vi "LiveVideo.vi"() -> ()   [LabVIEW 2019]
uses:
  <vilib>/userDefined/High Color/IMAQdx.ctl
  <vilib>/vision/driver/NI_Vision_Acquisition_Software.lvlib
  <vilib>/vision/NI_Vision_Development_Module.lvlib
panel:
  in  "Draw50umCircleAtCenter":bool
  out "Gcode":string
  in  "GetGantryXYZ":bool
  out "Position_XYZ":string
  in  "Corsshair":bool=TRUE
  out "Blue":T1(plugin-control)
  out "Green":T1(plugin-control)
  out "Red":T1(plugin-control)
  out "error out":errorcluster
  in  "Stop Button":bool
  out "Image":T1(plugin-control)
  in  "error in (no error)":errorcluster
  in  "Camera":T2="cam1"
  in  "ImageName":string="name1"
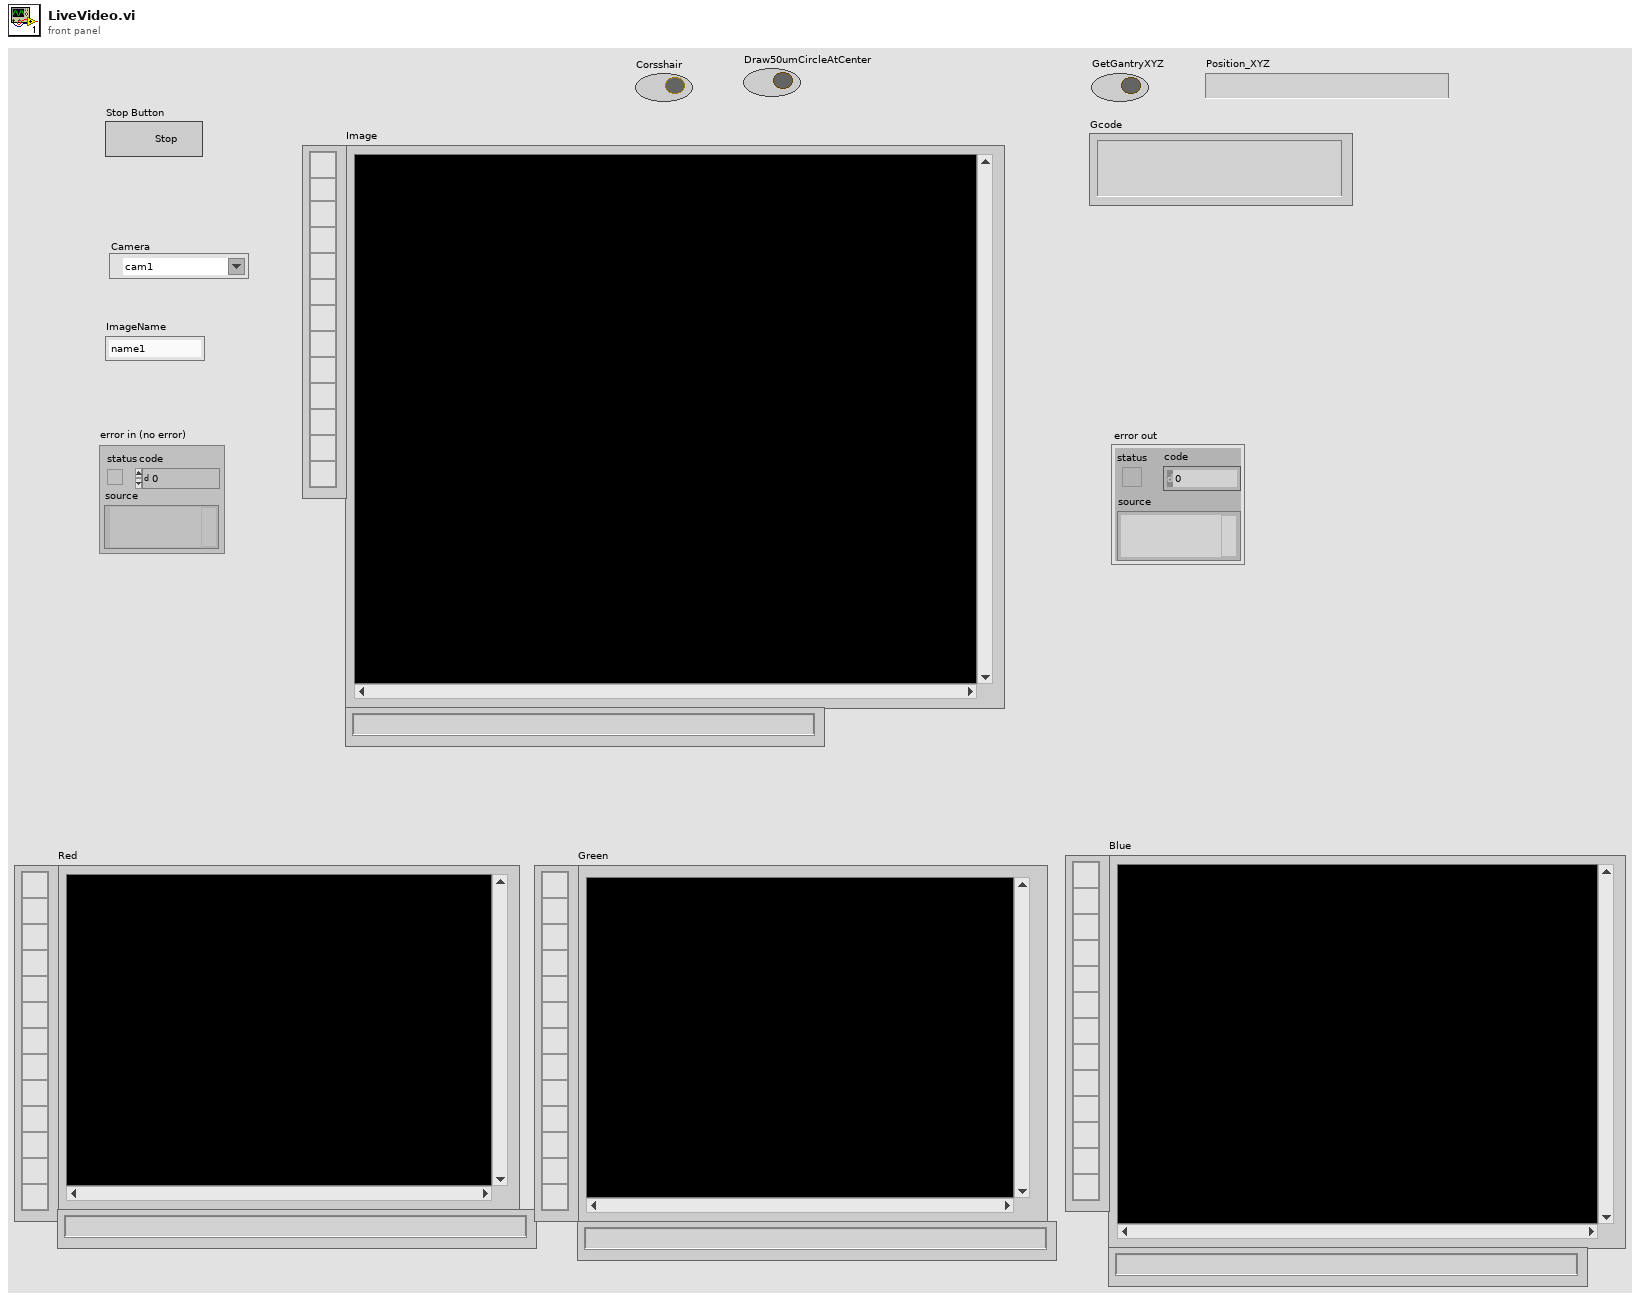
[diagram p1: front panel]
types:
  T1 = typedef "IMAQ Image.ctl" = refnum<image>
  T2 = typedef "IMAQdx.ctl" = refnum<k21>
  T3 = typedef "IMAQ Circle" = cluster{"Center X":i32, "Center Y":i32, "Inner Radius":i32, "Outer Radius":i32, "Start Angle":dbl, "End Angle":dbl}
  T4 = typedef "Image Type" = u32
  T5 = typedef "ROI Descriptor" = cluster{"Global Rectangle":i32[], "Contours":cluster{"ID":enum32{"External", "Internal"}, "Type":u32, "Coordinates":i32[]}[]}
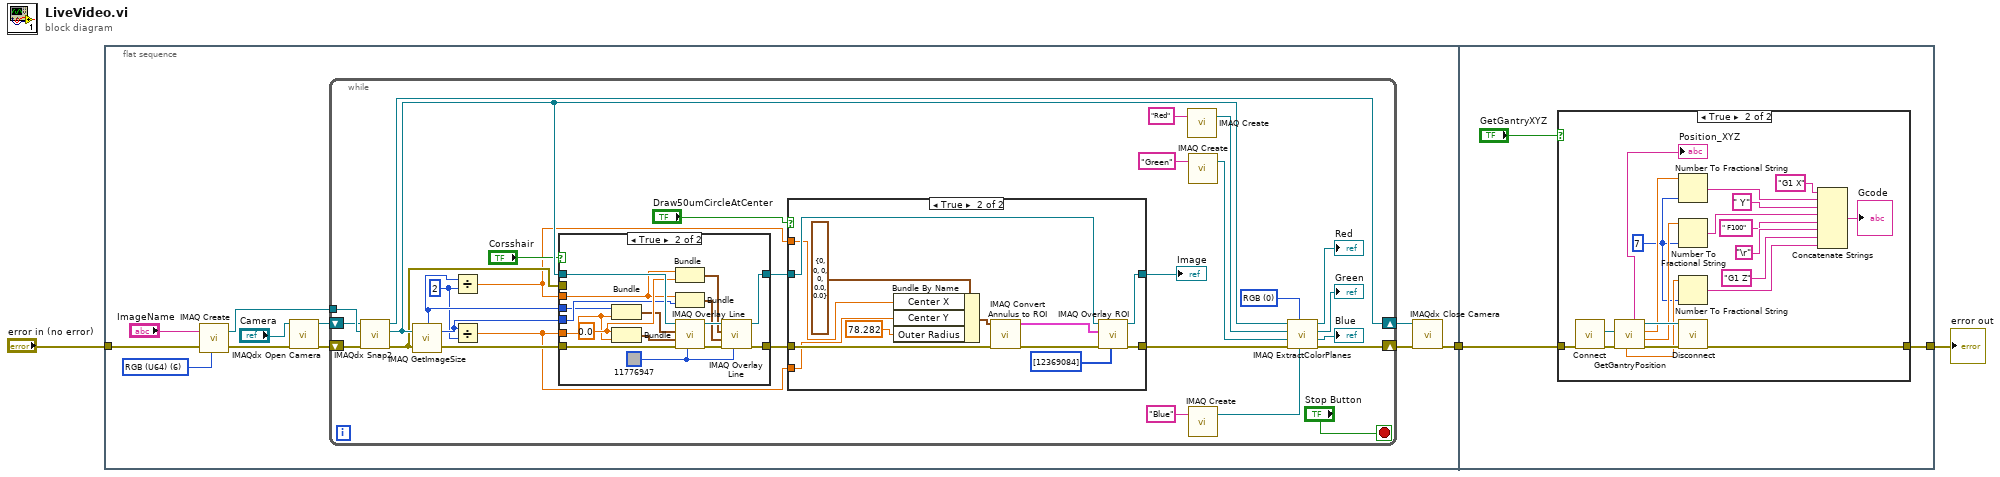
[diagram p0: block diagram]
diagram:
  n1 = flat-sequence {
    tunnel: "error in (no error)" -> [w10]
    tunnel: [w4] -> w2
    tunnel: w2 -> [w78]
    tunnel: [w77] -> w1
    frame #0 {
      w5 = T4 6 items=["Grayscale (U8)", "Grayscale (I16)", "Grayscale (SGL)", "Complex (CSG)", "RGB (U32)", "HSL (U32)", "RGB (U64)", "Grayscale (U16)"] ("Image Type")
      n2 = call "IMAQ Create"("Image Name"="ImageName", "Image Type"=w5, "error in (no error)"=w10) -> ("New Image"=w6:T1, "error out"=w7:errorcluster)  [unwired: 2 in]
      n3 = call <vilib>:"IMAQdx Open Camera.vi"("error in"=w7, "Session In"="Camera") -> ("error out"=w12:errorcluster, "Session Out"=w13:T2)  [unwired: 8 in]
      n4 = while {
        tunnel: w6 -> [w44]
        shift-right: [w27] -> w14
        shift-left: w12 -> [w42]
        shift-right: [w43] -> w11
        shift-left: w13 -> [w41]
        stop <- "Stop Button" stop-if-true
        w16 = 2 ("y")
        w38 = u16 0 items=["RGB", "HSL", "HSV", "HSI"] ("Color Mode")
        n5 = call <vilib>:"IMAQdx Snap2.vi"("error in"=w42, "Image In"=w44, "Session In"=w41) -> ("error out"=w28:errorcluster, "Image Out"=w29:T1, "Session Out"=w43:T2)  [unwired: 6 in]
        n6 = call "IMAQ GetImageSize"("Image"=w29, "error in (no error)"=w28) -> ("Y Resolution"=w20:i32, "X Resolution"=w19:i32, "error out"=w18:errorcluster)  [unwired: 2 in]
        n7 = Divide(x=w19, y=w16) -> (x/y=w15:dbl)
        n8 = Divide(x=w20, y=w16) -> (x/y=w17:dbl)
        n9 = case shown="True" "Corsshair" {
          tunnel: w29 -> [w60 w76]
          tunnel: w28 -> [w59 _]
          tunnel: [w60 w67] -> w25
          tunnel: [w59 w66] -> w24
          tunnel: w20 -> [_ w65]
          tunnel: w19 -> [_ w64]
          tunnel: w18 -> [_ w63]
          tunnel: w17 -> [_ w62]
          tunnel: w15 -> [_ w61]
          frame False {
          }
          frame True {
            w69 = u32 11776947 ("Color")
            w75 = 0.0 ("element")
            n10 = Bundle("X Resolution"=w64, w62) -> (w74:cluster{"X Resolution":i32, dbl})  [unwired: 1 in]
            n11 = Bundle("element"=w75, w62) -> (w73:cluster{"element":dbl, dbl})  [unwired: 1 in]
            n12 = Bundle(w61, "element"=w75) -> (w71:cluster{dbl, "element":dbl})  [unwired: 1 in]
            n13 = Bundle(w61, "Y Resolution"=w65) -> (w70:cluster{dbl, "Y Resolution":i32})  [unwired: 1 in]
            n14 = call "IMAQ Overlay Line"("Color"=w69, "error in (no error)"=w63, "End Point"=w73, "Start Point"=w74, "Image"=w76) -> ("error out"=w68:errorcluster, "Image Out"=w72:T1)  [unwired: 5 in]
            n15 = call "IMAQ Overlay Line"("Color"=w69, "error in (no error)"=w68, "End Point"=w70, "Start Point"=w71, "Image"=w72) -> ("error out"=w66:errorcluster, "Image Out"=w67:T1)  [unwired: 5 in]
          }
        }
        n16 = case shown="True" "Draw50umCircleAtCenter" {
          tunnel: w25 -> [w46 w53]
          tunnel: [w46 w52] -> w23
          tunnel: w24 -> [w45 w51]
          tunnel: [w45 w50] -> w22
          tunnel: w15 -> [_ w49]
          tunnel: w17 -> [_ w48]
          frame False {
          }
          frame True {
            n17 = Bundle By Name(cluster=T3 {"Center X"=0, "Center Y"=0, "Inner Radius"=0, "Outer Radius"=0, "Start Angle"=0.0, "End Angle"=0.0} ("Annulus"), "Center X"=w49, "Center Y"=w48, "Outer Radius"=78.282 ("CircleRadiusPixels")) -> (w58:T3)
            n18 = call "IMAQ Convert Annulus to ROI"("error in (no error)"=w51, "Annulus"=w58) -> ("error out"=w57:errorcluster, "ROI Descriptor"=w56:T5)  [unwired: 7 in]
            n19 = call "IMAQ Overlay ROI"("Colors (Green)"=u32[] [12369084], "error in (no error)"=w57, "ROI Descriptor"=w56, "Image"=w53) -> ("error out"=w50:errorcluster, "Image Out"=w52:T1)  [unwired: 6 in]
          }
        }
        "Image" <- w23
        n20 = call "IMAQ Create"("Image Name"="Red") -> ("New Image"=w37:T1)  [unwired: 3 in, 2 out]
        n21 = call "IMAQ Create"("Image Name"="Green") -> ("New Image"=w34:T1)  [unwired: 3 in, 2 out]
        n22 = call "IMAQ Create"("Image Name"="Blue") -> ("New Image"=w32:T1)  [unwired: 3 in, 2 out]
        n23 = call "IMAQ ExtractColorPlanes"("Blue or Luma or Val or Inten Plane"=w32, "Color Mode"=w38, "error in (no error)"=w22, "Green or Sat Plane"=w34, "Red or Hue Plane"=w37, "Image Src"=w29) -> ("error out"=w27:errorcluster, "Blue or Luma or Val or Inten Plane out"=→"Blue":T1, "Green or Sat Plane out"=→"Green":T1, "Red or Hue Plane out"=→"Red":T1)  [unwired: 2 in]
      }
      n24 = call <vilib>:"IMAQdx Close Camera.vi"("error in"=w14, "Session In"=w11) -> ("error out"=w4:errorcluster)  [unwired: 9 in]
    }
    frame #1 {
      n25 = case shown="True" "GetGantryXYZ" {
        tunnel: w78 -> [w80 w83]
        tunnel: [w80 w82] -> w77
        frame False {
        }
        frame True {
          w92 = i16 7 ("precision (6)")
          n26 = call "Connect.vi"("error in (no error)"=w83) -> ("error out"=w98:errorcluster, "controller"=w99:refnum<k24>)  [unwired: 9 in]
          n27 = call "GetGantryPosition.vi"("error in (no error)"=w98, "Controller In"=w99) -> ("error out"=w97:errorcluster, "Position Y"=w94:dbl, "Position X"=w95:dbl, "controller out"=w96:refnum<k24>, "Position_XYZ"=→"Position_XYZ":string, "Position Z"=w93:dbl)  [unwired: 3 in, 1 out]
          n28 = Number To Fractional String(number=w95, precision (6)=w92) -> (F-format string=w90:string)  [unwired: 2 in]
          n29 = Number To Fractional String(number=w94, precision (6)=w92) -> (F-format string=w88:string)  [unwired: 2 in]
          n30 = Number To Fractional String(number=w93, precision (6)=w92) -> (F-format string=w85:string)  [unwired: 2 in]
          n31 = call "Disconnect.vi"("error in (no error)"=w97, "controller"=w96) -> ("error out"=w82:errorcluster)  [unwired: 9 in]
          n32 = Concatenate Strings("G1 X" ("string"), w90, " Y" ("string"), w88, " F100" ("string"), "\r", "G1 Z" ("string"), w85) -> (→"Gcode":string)
        }
      }
    }
  }
  "error out" <- w1
